vi "Pre Launch Init.vi"(11 "Controller in":refnum<class "Controller.lvclass">) -> (0 "error out":errorcluster, 3 "Controller out":refnum<class "Controller.lvclass">)   [LabVIEW 2014, in "Controller.lvlib" / "Controller.lvclass"]
doc: "The <b>Controller::Pre Launch Init</b> reads data from the configuration file concerning the"
uses:
  Controller.lvclass
  Controls/Notifier Enum.ctl
  reusable/Switch/Switch.lvclass
  Messages/Update Filter State Params/Update Filter Cycle Params MSG.lvclass
  Messages/Change Filter State/Change Filter State.lvclass
  reusable/Session APIs/Session Log/System Log.lvclass
  Messages/Change Inlet MSG/Change Inlet MSG.lvclass
  reusable/Session APIs/File Access/Config Data/Config Data.lvclass
  reusable/Session APIs/File Access/Config Data/Config Data.lvclass/Config Data.ctl
  Controller.lvclass/Controller.ctl
  <vilib>/ActorFramework/Actor/Actor.lvclass/Actor.ctl
  <vilib>/ActorFramework/Message Enqueuer/Message Enqueuer.lvclass/Message Enqueuer.ctl
  Messages/Update Filter State Params/Update Filter Cycle Params MSG.lvclass/Update Filter Cycle Params MSG.ctl
  Messages/Update Switch State MSG/Update Switch MSG.lvclass/Update Switch MSG.ctl
  reusable/Session APIs/Session Log/System Log.lvclass/System Log.ctl
  Messages/Update Filter State Params/Write Period.vi
  Messages/Update Filter State Params/Write Length.vi
  Messages/Update Filter State Params/Write Cycle_.vi
  reusable/Session APIs/Session Log/Accessors/Write Main Path.vi
  reusable/Session APIs/Session Log/Accessors/Write Log Warnings_.vi
  reusable/Session APIs/Session Log/Accessors/Write Codes.vi
  reusable/Session APIs/File Access/Config Data/Accessors/Write Cfg Path.vi
  reusable/Session APIs/File Access/Config Data/Accessors/Read Ref.vi
  Messages/Update Switch State MSG/Write Val.vi
  <vilib>/ActorFramework/Message Enqueuer/Init from Existing Queue.vi
  <vilib>/ActorFramework/Message Priority Queue/Priority Enqueue.vi
  <vilib>/Utility/config.llb/Read Key (String).vi
  <vilib>/Utility/config.llb/Read Key (Boolean).vi
  <vilib>/Utility/config.llb/Read Key (I32).vi
  xGlobal Data.vi
  <vilib>/ActorFramework/Message Enqueuer/Message Enqueuer.lvclass
  <vilib>/ActorFramework/Actor/Actor.lvclass
  <vilib>/Utility/config.llb/NI_LVConfig.lvlib
  <vilib>/NI_Real-Time Target Support.lvlib
  <userlib>/_Session Fwk/Session - Root.lvclass
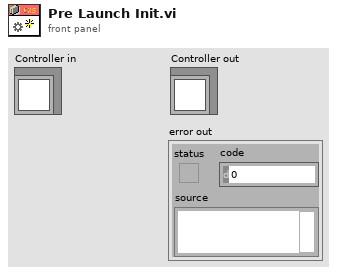
[diagram p1: front panel]
types:
  T1 = typedef "Notifier Enum.ctl" = enum16{"Initialize", "Get", "Set", "Close"}
  T2 = typedef "Session - Root.lvclass/Session Handle.ctl" = refnum<data-value>
  T3 = typedef "NI_LVConfig.lvlib/Config Data RefNum.ctl" = refnum<k1>
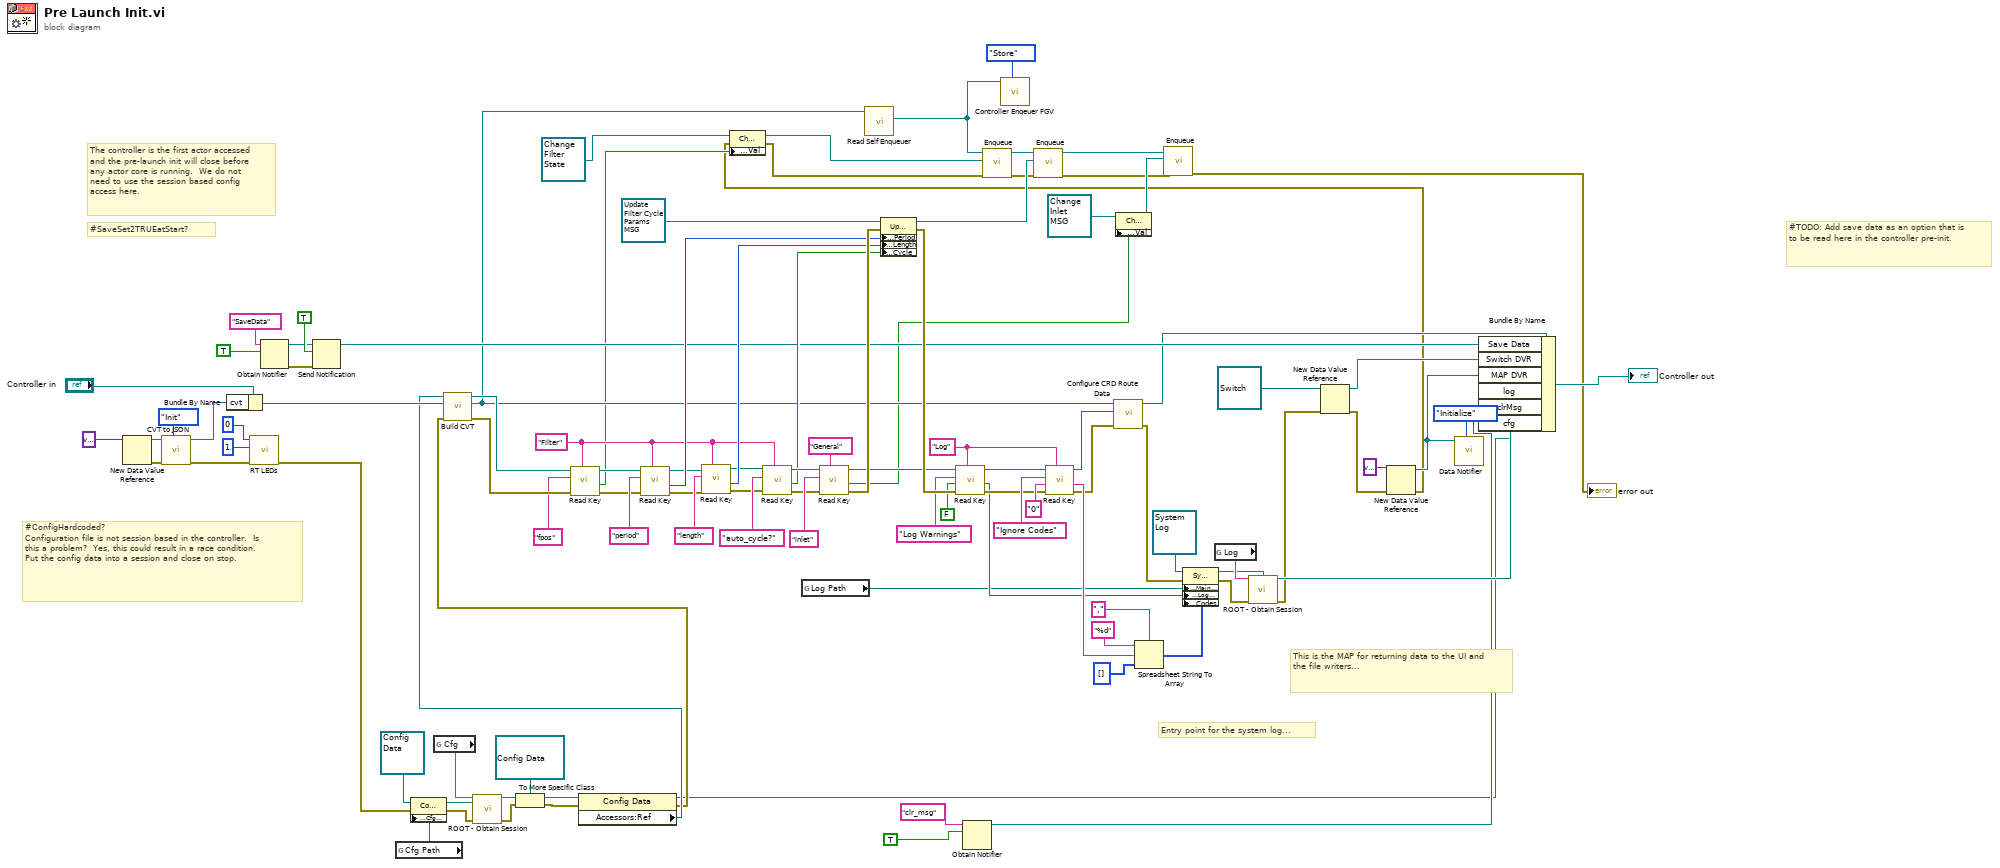
[diagram p0: block diagram]
diagram:
  w96 = "Log" ("section")
  w64 = "Filter" ("section")
  # "Entry point for the system log..."
  # "This is the MAP for returning data to the UI and the file writers..."
  # "#ConfigHardcoded?\nConfiguration file is not session based in the controller.  Is this a problem?  Yes, this could result in a race condition.  Put the config data into a session and close on stop."
  # "#SaveSet2TRUEatStart?"
  # "The controller is the first actor accessed and the pre-launch init will close before any actor core is running.  We do not need to use the session based config access here."
  # "#TODO: Add save data as an option that is to be read here in the controller pre-init."
  n1 = New Data Value Reference(data value=variant) -> (data value reference=w32:refnum<data-value>, error out=w31:errorcluster)  [unwired: 1 in]
  n2 = call "CVT to JSON.vi"("Select"=enum16{"Init", "Get", "Destroy"}."Init", "error in"=w31, "cvt in"=w32) -> ("error out"=w27:errorcluster, "cvt out"=w29:refnum<data-value>)  [unwired: 6 in, 1 out]
  n3 = Bundle By Name(cluster="Controller in", "cvt"=w29) -> (w28:refnum<class "Controller.lvclass">)
  n4 = call <vilib>:"RT LEDs.vi"("error in (no error)"=w27, "State"=1, "LED Num"=0) -> ("error out"=w18:errorcluster)  [unwired: 3 in, 1 out]
  n5 = Obtain Notifier(name (unnamed)="SaveData", notification data type=TRUE) -> (notifier out=w47:refnum<notifier>, error out=w48:errorcluster)  [unwired: 2 in, 1 out]
  n6 = Send Notification(notification=TRUE, notifier=w47, error in (no error)=w48) -> (notifier out=w50:refnum<notifier>)  [unwired: 1 out]
  n7 = global read "xGlobal Data.vi" "Cfg Path"() -> (w21:path)
  n8 = property class="Config Data"(reference=refnum<class "Config Data.lvclass"> refnum ("Config Data"), error in=w18, "Accessors:Cfg Path"=w21) -> (reference out=w20:refnum<class "Config Data.lvclass">, error out=w19:errorcluster)
  n9 = global read "xGlobal Data.vi" "Cfg"() -> (w23:string)
  n10 = call <userlib>:"ROOT - Obtain Session.vi"("Session Name ()"=w23, "OBJ - Session"=w20, "error in (no error)"=w19) -> ("Session Handle"=w24:T2, "error out"=w25:errorcluster)  [unwired: 10 in, 1 out]
  n11 = To More Specific Class(target class=refnum<data-value> refnum ("Session Handle"), reference=w24, error in=w25) -> (specific class reference=w17:refnum<data-value>, error out=w16:errorcluster)
  n12 = property class="Config Data"(reference=w17, error in=w16) -> (reference out=w13:refnum<data-value>, error out=w14:errorcluster, "Accessors:Ref"=w15:T3)
  n13 = call "Build CVT.vi"("Error In"=w14, "Controller in"=w28, "CfgRef"=w15) -> ("Error Out"=w84:errorcluster, "Controller out"=w38:refnum<class "Controller.lvclass">, "refnum out"=w83:T3)  [unwired: 6 in]
  n14 = call-poly <vilib>:"Read Key.vi"("section"=w64, "error in (no error)"=w84, "key"="fpos", "refnum"=w83) -> ("error out"=w53:errorcluster, "value"=w12:bool, "refnum out"=w52:T3)  [unwired: 4 in, 1 out]
  n15 = call-poly <vilib>:"Read Key.vi"("section"=w64, "error in (no error)"=w53, "key"="period", "refnum"=w52) -> ("error out"=w56:errorcluster, "value"=w80:i32, "refnum out"=w55:T3)  [unwired: 4 in, 1 out]
  n16 = call-poly <vilib>:"Read Key.vi"("section"=w64, "error in (no error)"=w56, "key"="length", "refnum"=w55) -> ("error out"=w63:errorcluster, "value"=w81:i32, "refnum out"=w62:T3)  [unwired: 4 in, 1 out]
  n17 = call-poly <vilib>:"Read Key.vi"("section"=w64, "error in (no error)"=w63, "key"="auto_cycle?", "refnum"=w62) -> ("error out"=w86:errorcluster, "value"=w82:bool, "refnum out"=w85:T3)  [unwired: 4 in, 1 out]
  n18 = global read "xGlobal Data.vi" "Log Path"() -> (w78:path)
  n19 = call-poly <vilib>:"Read Key.vi"("section"="General", "error in (no error)"=w86, "key"="inlet", "refnum"=w85) -> ("error out"=w104:errorcluster, "value"=w7:bool, "refnum out"=w90:T3)  [unwired: 4 in, 1 out]
  n20 = call <vilib>:"Read Self Enqueuer.vi"("Actor"=w38) -> ("Self Enqueuer"=w68:refnum<class "Message Enqueuer.lvclass">)  [unwired: 10 in]
  n21 = property class="Update Filter Cycle Params"(reference=refnum<class "Update Filter Cycle Params MSG.lvclass"> refnum ("Controller.lvlib:Update Filter Cycle Params"), error in=w104, "Accessors:Period"=w80, "Accessors:Length"=w81, "Accessors:Cycle_"=w82) -> (reference out=w70:refnum<class "Update Filter Cycle Params MSG.lvclass">, error out=w105:errorcluster)
  n22 = call-poly <vilib>:"Read Key.vi"("section"=w96, "error in (no error)"=w105, "default value"=FALSE, "key"="Log Warnings", "refnum"=w90) -> ("error out"=w95:errorcluster, "value"=w93:bool, "refnum out"=w94:T3)  [unwired: 3 in, 1 out]
  n23 = Obtain Notifier(name (unnamed)="clr_msg", notification data type=TRUE) -> (notifier out=w41:refnum<notifier>)  [unwired: 2 in, 2 out]
  n24 = call "Controller Enqeuer FGV.vi"("State"=enum16{"Store", "Send MSG"}."Store", "Enqueuer"=w68) -> ()  [unwired: 9 in, 1 out]
  n25 = call-poly <vilib>:"Read Key.vi"("section"=w96, "error in (no error)"=w95, "default value"="0", "key"="Ignore Codes", "refnum"=w94) -> ("error out"=w37:errorcluster, "value"=w99:string, "refnum out"=w39:T3)  [unwired: 3 in, 1 out]
  n26 = call "Configure CRD Route Data.vi"("error in"=w37, "CfgRefIn"=w39, "Controller in"=w38) -> ("error out"=w36:errorcluster, "Controller out"=w35:refnum<class "Controller.lvclass">)  [unwired: 6 in, 1 out]
  n27 = property class="Change Inlet MSG.lvclass"(reference=refnum<class "Change Inlet MSG.lvclass"> refnum ("Controller.lvlib:Change Inlet MSG.lvclass"), "Accessors:Val"=w7) -> (reference out=w8:refnum<class "Change Inlet MSG.lvclass">)  [unwired: 1 in, 1 out]
  n28 = Spreadsheet String To Array(delimiter (Tab)=",", format string="%d", spreadsheet string=w99, array type (2D Dbl)=i32[] []) -> (array=w103:i32[])
  n29 = property class="Sys Log"(reference=refnum<class "System Log.lvclass"> refnum ("Sys Log"), error in=w36, "Accessors:Main Path"=w78, "Accessors:Log Warnings_"=w93, "Accessors:Codes"=w103) -> (reference out=w76:refnum<class "System Log.lvclass">, error out=w74:errorcluster)
  n30 = global read "xGlobal Data.vi" "Log"() -> (w77:string)
  n31 = call <userlib>:"ROOT - Obtain Session.vi"("Session Name ()"=w77, "OBJ - Session"=w76, "error in (no error)"=w74) -> ("Session Handle"=w79:T2, "error out"=w4:errorcluster)  [unwired: 10 in, 1 out]
  n32 = New Data Value Reference(data value=refnum<class "Switch.lvclass"> refnum ("Switch"), error in=w4) -> (data value reference=w71:refnum<data-value>, error out=w60:errorcluster)
  n33 = New Data Value Reference(data value=variant, error in=w60) -> (data value reference=w72:refnum<data-value>, error out=w3:errorcluster)
  n34 = property class="Change Filter State MSG"(reference=refnum<class "Change Filter State.lvclass"> refnum ("Controller.lvlib:Change Filter State MSG"), error in=w3, "Accessors:Val"=w12) -> (reference out=w10:refnum<class "Change Filter State.lvclass">, error out=w2:errorcluster)
  n35 = call <vilib>:"Enqueue.vi"("error in (no error)"=w2, "Message"=w10, "Message Enqueuer in"=w68) -> ("error out"=w6:errorcluster, "Message Enqueuer out"=w69:refnum<class "Message Enqueuer.lvclass">)  [unwired: 7 in]
  n36 = call <vilib>:"Enqueue.vi"("error in (no error)"=w6, "Message"=w70, "Message Enqueuer in"=w69) -> ("error out"=w5:errorcluster, "Message Enqueuer out"=w89:refnum<class "Message Enqueuer.lvclass">)  [unwired: 7 in]
  n37 = call <vilib>:"Enqueue.vi"("error in (no error)"=w5, "Message"=w8, "Message Enqueuer in"=w89) -> ("error out"=→"error out":errorcluster)  [unwired: 7 in, 1 out]
  n38 = call "Data Notifier.vi"("State"=Notifier_Enum."Initialize", "MAP DVR"=w72) -> ()  [unwired: 8 in, 2 out]
  n39 = Bundle By Name(cluster=w35, "Save Data"=w50, "Switch DVR"=w71, "MAP DVR"=w72, "log"=w79, "clrMsg"=w41, "cfg"=w13) -> (→"Controller out":refnum<class "Controller.lvclass">)
